vi "WaveformCheck.vi"(8 "error in (no error)":errorcluster, 11 "Class In":refnum<class "ScopePluginsBase.lvclass">) -> (0 "error out":errorcluster, 1 "Run?":bool, 2 "Continuous":bool, 3 "Class Out":refnum<class "ScopePluginsBase.lvclass">)   [LabVIEW 2018, in "ScopePlugins.lvlib"]
uses:
  ScopePlugins.lvlib
  ScopePluginBaseClass/ScopePluginsBase.lvclass
  ScopePluginBaseClass/ScopePluginsBase.lvclass/ScopePluginsBase.ctl
  ScopePluginBaseClass/Accessors/Read Channels.vi
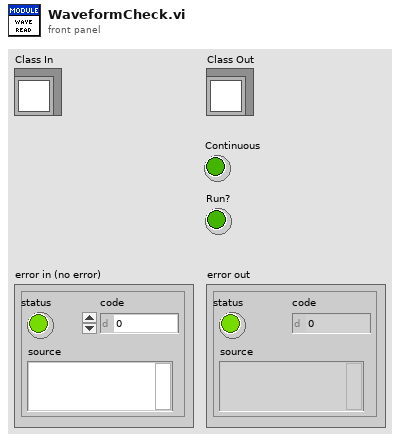
[diagram p1: front panel]
types:
  T1 = typedef "ScopePlugins.lvlib/ScopePluginsBase.lvclass/ChannelSetting(s).ctl" = cluster{"Number of Channels":i32, "Channel(s)":cluster{"Enabled":bool, "Instrument Handle":string, "Channel Name":string, "Maximum Input Frequency":dbl, "Verticle Settings":cluster{"Vertical Range":dbl, "Vertical Offset":dbl, "Probe Attenuation":dbl, "Vertical Coupling":i32}, "Connected":bool, "Input Impedance":dbl, "IO Type Instrument Handle":refnum<k15>}[]}
  T2 = typedef "ScopePlugins.lvlib/ScopePluginsBase.lvclass/HorizontalSettings.ctl" = cluster{"Continuous":bool, "EnableAveraging":bool, "Number Averages":i32, "Measurement Timeout":dbl, "Min Record Length":i32, "Min Sample Rate":dbl, "Enforce Realtime":bool, "Sampling Mode ":enum16{"Real Time", "Equivalent Time", "Segment", "Real Time Peak Detect", "Real Time High Resolution", "Peak Detect Segment", "High Resolution Segment"}, "Interpolation":enum16{"No Interpolation", "sin(x)/x", "linear", "1 Point sin(x)/x", "2 Point sin(x)/x", "4 Point sin(x)/x", "8 Point sin(x)/x", "16 Point sin(x)/x"}, "Type":enum16{"Normal", "PeakDetect", "HighRes", "Envelope", "Average"}, "StartTime":dbl, "Time Per Record":dbl, "Number of Points Minimum":i32, "Measurement Name":string, "Measurement RefreshTime (ms)":u32}
  T3 = cluster{"Enabled":bool, "Instrument Handle":string, "Channel Name":string, "Maximum Input Frequency":dbl, "Verticle Settings":cluster{"Vertical Range":dbl, "Vertical Offset":dbl, "Probe Attenuation":dbl, "Vertical Coupling":i32}, "Connected":bool, "Input Impedance":dbl, "IO Type Instrument Handle":refnum<k15>}[]
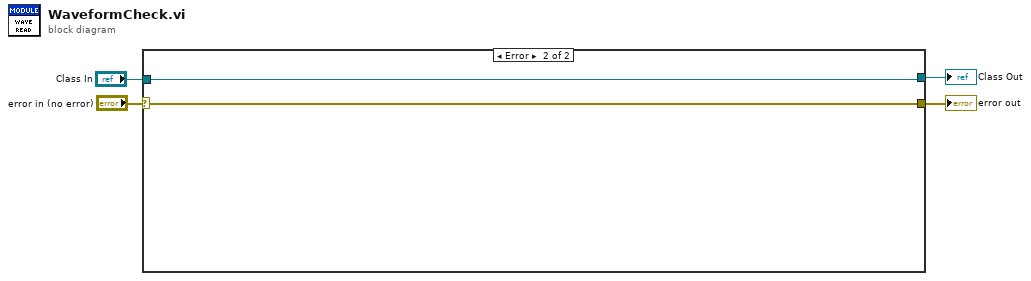
[diagram p0: block diagram]
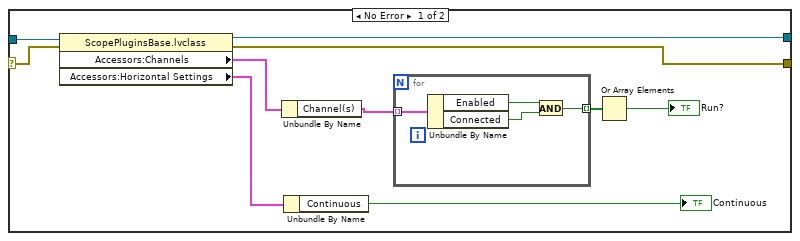
[diagram p2: hidden frame]
diagram:
  n1 = case shown="Error" "error in (no error)" {
    selector: "error in (no error)" -> [w10 w19]
    tunnel: "Class In" -> [w11 w20]
    tunnel: [w9 w20] -> w2
    tunnel: [w8 w19] -> w1
    frame No Error {
      n2 = property class="ScopePluginsBase.lvclass"(reference=w11, error in=w10) -> (reference out=w9:refnum<class "ScopePluginsBase.lvclass">, error out=w8:errorcluster, "Accessors:Channels"=w12:T1, "Accessors:Horizontal Settings"=w5:T2)
      n3 = Unbundle By Name(w12) -> ("Channel(s)"=w14:T3)
      n4 = Unbundle By Name(w5) -> ("Continuous"=→"Continuous":bool)
      n5 = for {
        tunnel: w14 -> [w18] mode=indexing
        tunnel: [w15] -> w13 mode=indexing
        n6 = Unbundle By Name(w18) -> ("Enabled"=w17:bool, "Connected"=w16:bool)
        n7 = And(x=w17, y=w16) -> (x .and. y?=w15:bool)
      }
      n8 = Or Array Elements(Boolean array=w13) -> (logical OR=→"Run?":bool)
    }
    frame Error {
    }
  }
  "error out" <- w1
  "Class Out" <- w2
